vi "Get XY Plot Properties from Graph.vi"(8 "error in (no error)":errorcluster, 11 "Graph":refnum<vi>) -> (0 "error out":errorcluster, 3 "Plots":T1[](array[typedef]), 5 "Legend:Number of Rows":u32)   [LabVIEW 2013, in "Workspace MultiY Graph.lvlib"]
uses:
  Workspace MultiY Graph.lvlib
  XY Plot Properties.ctl
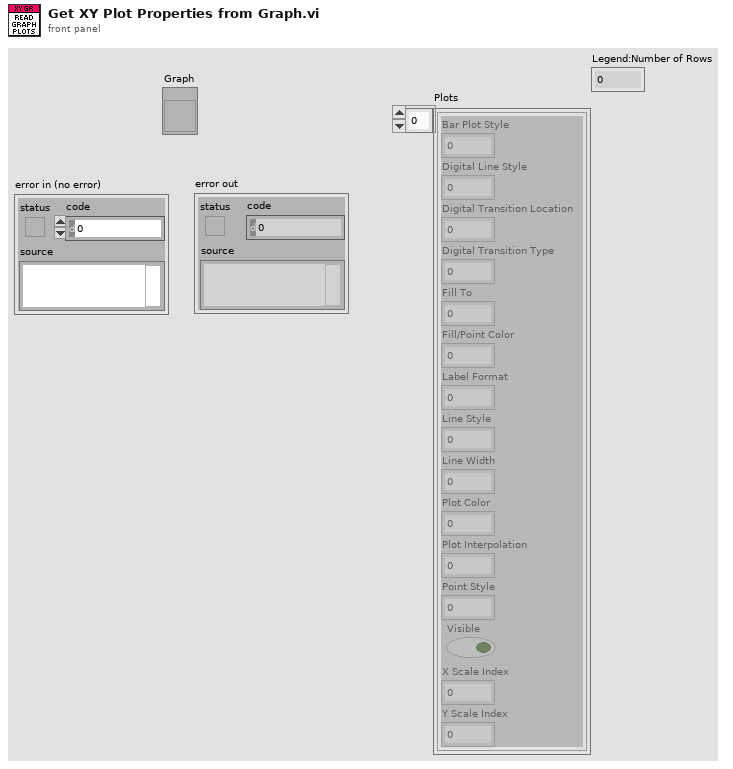
[diagram p1: front panel]
types:
  T1 = typedef "Workspace MultiY Graph.lvlib/XY Plot Properties.ctl" = cluster{"Bar Plot Style":u8, "Digital Line Style":u8, "Digital Transition Location":u8, "Digital Transition Type":u8, "Fill To":i16, "Fill/Point Color":u32, "Label Format":u8, "Line Style":u8, "Line Width":u8, "Plot Color":u32, "Plot Interpolation":u8, "Point Style":u8, "Visible":bool, "X Scale Index":u32, "Y Scale Index":u32}
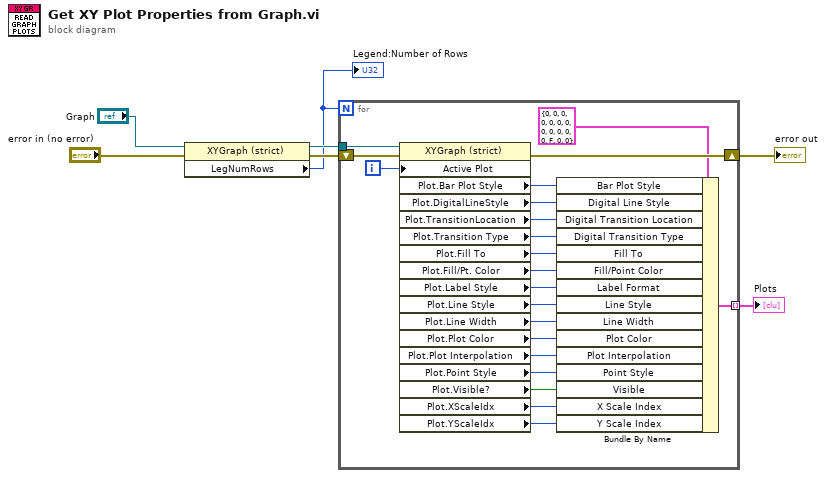
[diagram p0: block diagram]
diagram:
  n1 = property class="XYGraph (strict)"(reference="Graph", error in="error in (no error)") -> (reference out=w4:refnum<vi>, error out=w5:errorcluster, "LegNumRows"=w3:u32)
  "Legend:Number of Rows" <- w3
  n2 = for {
    N: w3 -> [_]
    shift-right: [w25] -> w7
    shift-left: w5 -> [w28]
    tunnel: w4 -> [w27]
    tunnel: [w8] -> w2 mode=indexing
    i -> [w26]
    n3 = property class="XYGraph (strict)"(reference=w27, error in=w28, "Active Plot"=w26) -> (error out=w25:errorcluster, "Plot.Bar Plot Style"=w23:u8, "Plot.DigitalLineStyle"=w22:u8, "Plot.TransitionLocation"=w21:u8, "Plot.Transition Type"=w20:u8, "Plot.Fill To"=w19:i16, "Plot.Fill/Pt. Color"=w18:u32, "Plot.Label Style"=w17:u8, "Plot.Line Style"=w16:u8, "Plot.Line Width"=w15:u8, "Plot.Plot Color"=w14:u32, "Plot.Plot Interpolation"=w13:u8, "Plot.Point Style"=w12:u8, "Plot.Visible?"=w11:bool, "Plot.XScaleIdx"=w10:u32, "Plot.YScaleIdx"=w9:u32)  [unwired: 1 out]
    n4 = Bundle By Name(cluster=T1 {"Bar Plot Style"=0, "Digital Line Style"=0, "Digital Transition Location"=0, "Digital Transition Type"=0, "Fill To"=0, "Fill/Point Color"=0, "Label Format"=0, "Line Style"=0, "Line Width"=0, "Plot Color"=0, "Plot Interpolation"=0, "Point Style"=0, "Visible"=FALSE, "X Scale Index"=0, "Y Scale Index"=0} ("Plot Props"), "Bar Plot Style"=w23, "Digital Line Style"=w22, "Digital Transition Location"=w21, "Digital Transition Type"=w20, "Fill To"=w19, "Fill/Point Color"=w18, "Label Format"=w17, "Line Style"=w16, "Line Width"=w15, "Plot Color"=w14, "Plot Interpolation"=w13, "Point Style"=w12, "Visible"=w11, "X Scale Index"=w10, "Y Scale Index"=w9) -> (w8:T1)
  }
  "error out" <- w7
  "Plots" <- w2
